vi "Draw.vi"(8 "error in (no error)":errorcluster, 9 "disable contained items?":bool, 10 "IB_Tree":refnum<class "IB_Tree.lvclass">, 11 "IB_TreeContainerItem in":refnum<class "IB_Tree_Item_Source_Container.lvclass">) -> (0 "error out":errorcluster, 3 "IB_TreeContainerItem out":refnum<class "IB_Tree_Item_Source_Container.lvclass">)   [LabVIEW 2020, in "IB_Tree_Item_Source_Container.lvclass"]
uses:
  <vilib>/AppBuilder/IB_Classes/Tree_Item_Source_Container/IB_Tree_Item_Source_Container.lvclass
  <vilib>/AppBuilder/IB_Classes/Tree_Item_Source_Container/IB_Tree_Item_Source_Container.lvclass/IB_Tree_Item_Source_Container.ctl
  <vilib>/AppBuilder/IB_Classes/Tree_Item_Source/IB_Tree_Item_Source.lvclass
  <vilib>/AppBuilder/IB_Classes/Tree_Item_Source_Contained_File/IB_Tree_Item_Source_Contained_File.lvclass
  <vilib>/AppBuilder/IB_Classes/Tree/IB_Tree.lvclass
  e:/builds/penguin/labview/branches/2020/dev/dist/vi.lib/AppBuilder/IB_Classes/Tree_Item_Source/IB_Tree_Item_Source.lvclass
  e:/builds/penguin/labview/branches/2020/dev/dist/vi.lib/AppBuilder/IB_Classes/Tree_Item/IB_Tree_Item.lvclass
  e:/builds/penguin/labview/branches/2020/dev/dist/vi.lib/AppBuilder/IB_Classes/Tree_Item_Source_Container/IB_Tree_Item_Source_Container.lvclass
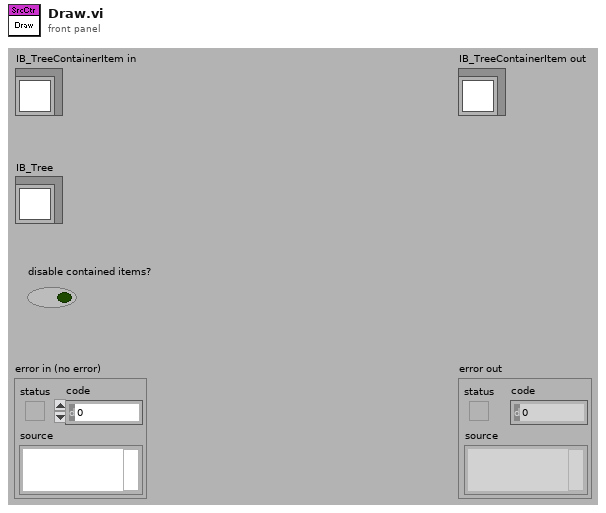
[diagram p1: front panel]
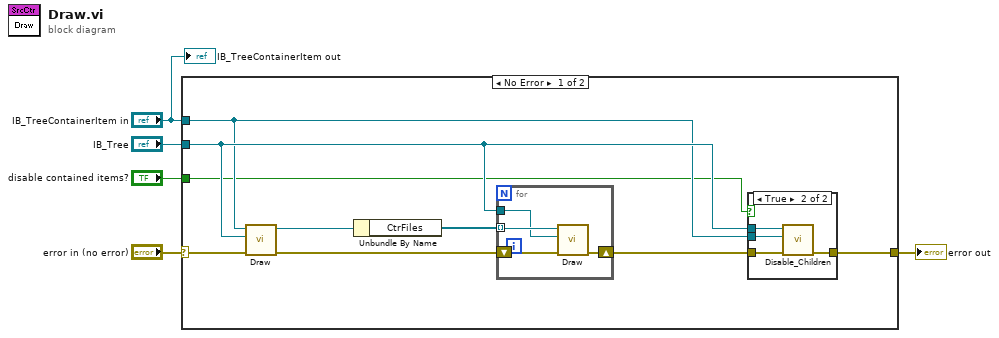
[diagram p0: block diagram]
diagram:
  n1 = case shown="No Error" "error in (no error)" {
    selector: "error in (no error)" -> [w14 w24]
    tunnel: [w9 w24] -> w5
    tunnel: "IB_Tree" -> [w11 _]
    tunnel: "IB_TreeContainerItem in" -> [w8 _]
    tunnel: "disable contained items?" -> [w6 _]
    frame No Error {
      n2 = call-parent "Draw.vi"("error in (no error)"=w14, "IB_Tree"=w11, "IB_TreeItem in"=w8) -> ("error out"=w12:errorcluster, "IB_TreeItem out"=w7:refnum<class "IB_Tree_Item_Source_Container.lvclass">)  [unwired: 1 in, 6 out]
      n3 = Unbundle By Name(w7) -> ("CtrFiles"=w13:refnum<class "IB_Tree_Item_Source_Contained_File.lvclass">[])
      n4 = for {
        tunnel: w13 -> [w23] mode=indexing
        tunnel: w11 -> [w22]
        shift-right: [w20] -> w10
        shift-left: w12 -> [w21]
        n5 = call-dynamic "Draw.vi"("error in (no error)"=w21, "IB_Tree"=w22, "IB_TreeCtrFileItem in"=w23) -> ("error out"=w20:errorcluster)  [unwired: 1 in, 7 out]
      }
      n6 = case shown="True" w6 {
        tunnel: w11 -> [_ w19]
        tunnel: w10 -> [w15 w18]
        tunnel: [w15 w17] -> w9
        tunnel: w8 -> [_ w16]
        frame False {
        }
        frame True {
          n7 = call <vilib>:"Disable_Children.vi"("error in (no error)"=w18, "Tree item"=w16, "IB_Tree in"=w19) -> ("error out"=w17:errorcluster)  [unwired: 8 out]
        }
      }
    }
    frame Error {
    }
  }
  "error out" <- w5
  "IB_TreeContainerItem out" <- "IB_TreeContainerItem in"
